vi "Drive Problem Fix.vi"(1 "Drive Global Data Modified":T1, 2 "Drive Global Data Original":T1) -> (0 "Drive Global Data New":T1)   [LabVIEW 2013]
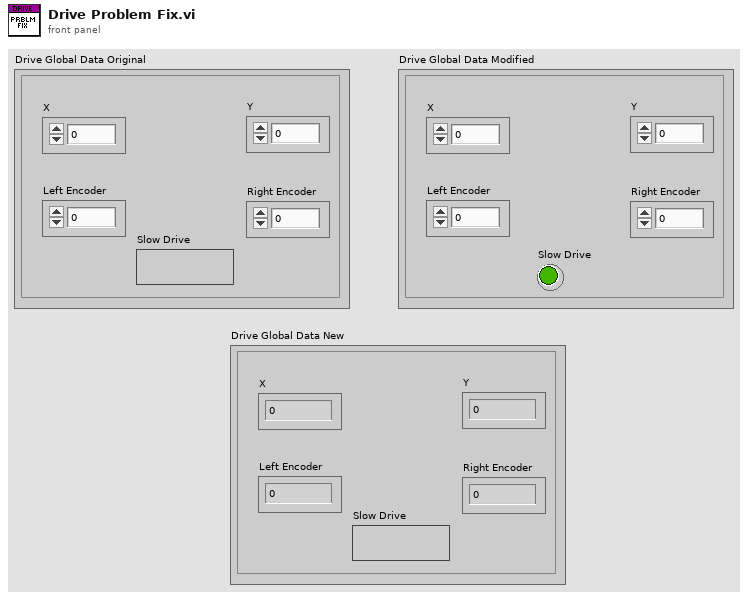
[diagram p1: front panel]
types:
  T1 = cluster{"Y":dbl, "X":dbl, "Left Encoder":dbl, "Right Encoder":dbl, "Slow Drive":bool}
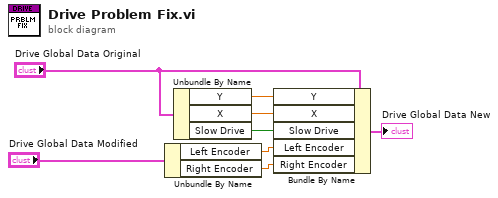
[diagram p0: block diagram]
diagram:
  n1 = Unbundle By Name("Drive Global Data Modified") -> ("Left Encoder"=w2:dbl, "Right Encoder"=w1:dbl)
  n2 = Unbundle By Name("Drive Global Data Original") -> ("Y"=w6:dbl, "X"=w5:dbl, "Slow Drive"=w3:bool)
  n3 = Bundle By Name(cluster="Drive Global Data Original", "Y"=w6, "X"=w5, "Slow Drive"=w3, "Left Encoder"=w2, "Right Encoder"=w1) -> (→"Drive Global Data New":T1)
